vi "Module Launcher.vi"   [LabVIEW 2014]
uses:
  User Event/User Event Action.ctl
  User Module/User Module.lvlib
  Display Module/Display Module.lvlib
  Control Module/Control Module.lvlib
  Error Module/Error Module.lvlib
  Sensor Module/Sensor Module.lvlib
  Database Module/Database Module.lvlib
types:
  T1 = typedef "User Event Action.ctl" = enum16{"Get", "Create", "Destroy"}
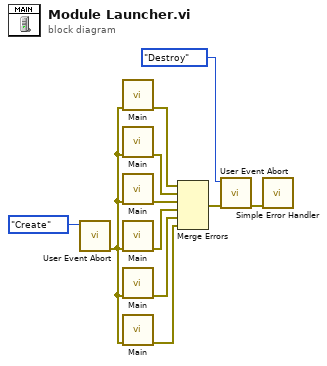
[diagram p0: block diagram]
diagram:
  n1 = call "User Event Abort.vi"("Action"=User_Event_Action."Create") -> ("error out"=w10:errorcluster)  [unwired: 9 in, 1 out]
  n2 = call "Main.vi"("error in (no error)"=w10) -> ("error out"=w9:errorcluster)  [unwired: 10 in]
  n3 = call "Main.vi"("error in (no error)"=w10) -> ("error out"=w8:errorcluster)  [unwired: 10 in]
  n4 = call "Main.vi"("error in (no error)"=w10) -> ("error out"=w7:errorcluster)  [unwired: 10 in]
  n5 = call "Main.vi"("error in (no error)"=w10) -> ("error out"=w6:errorcluster)  [unwired: 10 in]
  n6 = call "Main.vi"("error in (no error)"=w10) -> ("error out"=w5:errorcluster)  [unwired: 10 in]
  n7 = call "Main.vi"("error in (no error)"=w10) -> ("error out"=w4:errorcluster)  [unwired: 10 in]
  n8 = Merge Errors(w9, w8, w7, w6, w5, w4) -> (w2:errorcluster)
  n9 = call "User Event Abort.vi"("error in (no error)"=w2, "Action"=User_Event_Action."Destroy") -> ("error out"=w1:errorcluster)  [unwired: 8 in, 1 out]
  n10 = call <vilib>:"Simple Error Handler.vi"("error in (no error)"=w1) -> ()  [unwired: 4 in, 5 out]
